vi "green_threshing.vi"(2 "lum":cluster{"Lower value":i32, "Upper value":i32}={"Lower value"=0, "Upper value"=255}, 4 "sat":cluster{"Lower value":i32, "Upper value":i32}={"Lower value"=0, "Upper value"=255}, 5 "hue":cluster{"Lower value":i32, "Upper value":i32}={"Lower value"=50, "Upper value"=102}, 6 "error in (no error)":errorcluster, 9 "Image Src":T1) -> (0 "error out":errorcluster, 1 "circular particles":dbl[][](array[numeric]), 3 "Image Out":T1(plugin-control))   [LabVIEW 2009]
uses:
  <vilib>/vision/Image Controls.llb/IMAQ Image.ctl
  <vilib>/vision/NI_Vision_Development_Module.lvlib
panel:
  in  "max circularity":dbl=1.095
  out "size(s)":i32[](array[numeric])
  out "Particle Measurements (Pixels)":dbl[][](array[numeric]) format="%.2f"
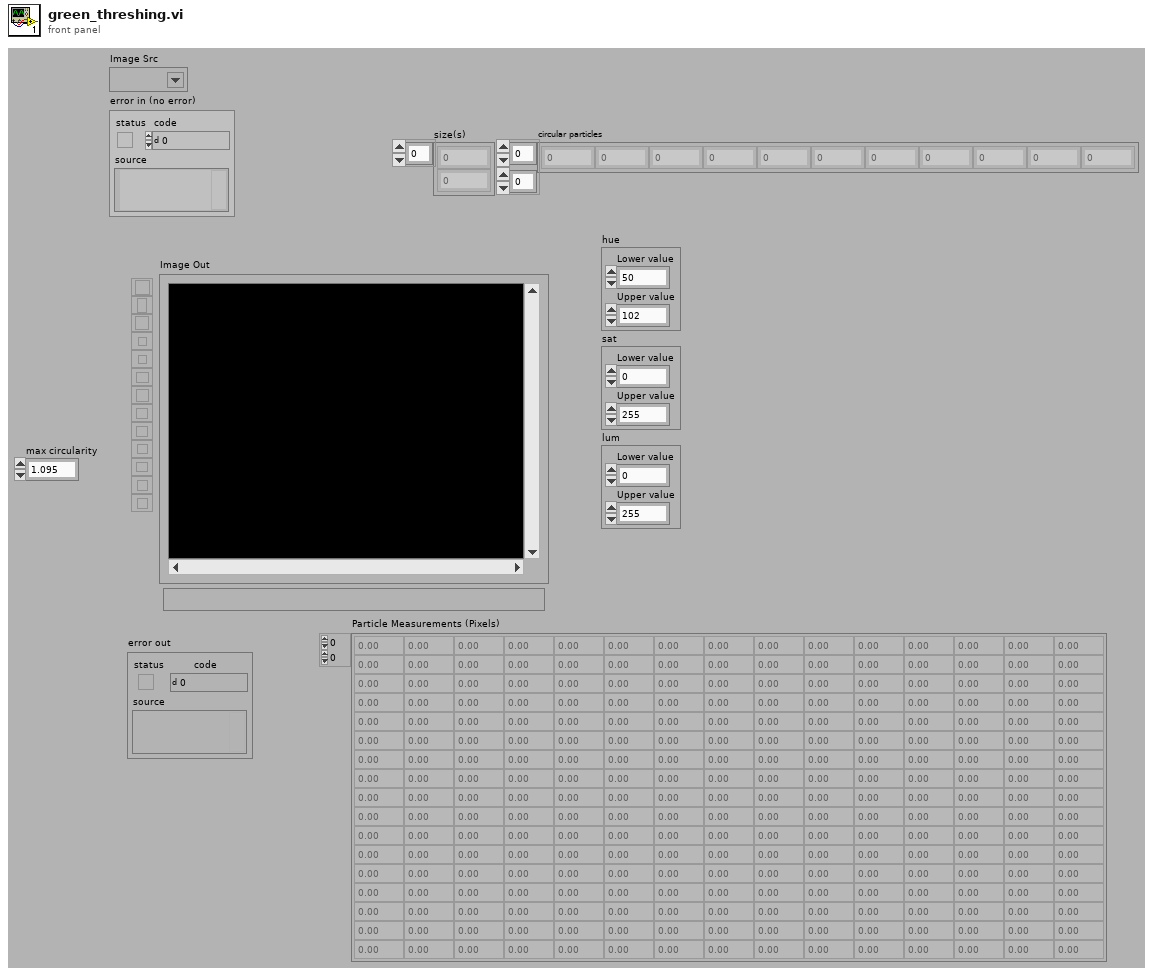
[diagram p1: front panel]
types:
  T1 = typedef "IMAQ Image.ctl" = refnum<image>
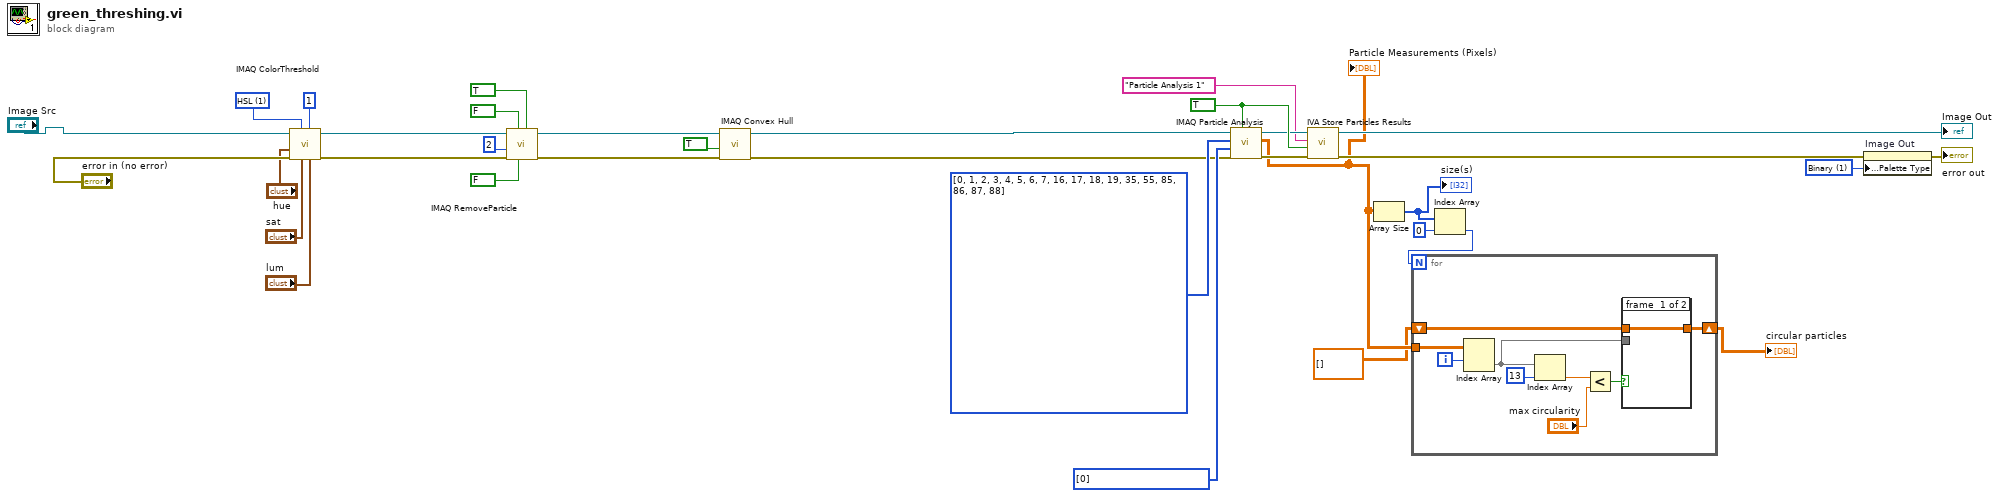
[diagram p0: block diagram]
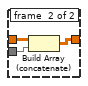
[diagram p2: hidden frame]
diagram:
  w16 = u16 1 items=["RGB", "HSL", "HSV", "HSI"] ("Color Mode")
  w27 = u32 1 items=["Grayscale", "Binary", "Gradient", "Rainbow", "Temperature", "User Defined"] ("Palette")
  w34 = i32[] [0] items=["Center of Mass X", "Center of Mass Y", "First Pixel X", "First Pixel Y", "Bounding Rect Left", "Bounding Rect Top", "Bounding Rect Right", "Bounding Rect Bottom", "Max Feret Diameter Start X", "Max Feret Diameter Start Y", "Max Feret Diameter End X", "Max Feret Diameter End Y", "Max Horiz. Segment Length Left", "Max Horiz. Segment Length Right", "Max Horiz. Segment Length Row", "-", "Bounding Rect Width", "Bounding Rect Height", "Bounding Rect Diagonal", "Perimeter", "Convex Hull Perimeter", "Holes' Perimeter", "Max Feret Diameter", "Equivalent Ellipse Major Axis", "Equivalent Ellipse Minor Axis", "Equivalent Ellipse Minor Axis (Feret)", "Equivalent Rect Long Side", "Equivalent Rect Short Side", "Equivalent Rect Diagonal", "Equivalent Rect Short Side (Feret)", "Average Horiz. Segment Length", "Average Vert. Segment Length", "Hydraulic Radius", "Waddel Disk Diameter", "-", "Area", "Holes' Area", "Particle & Holes' Area", "Convex Hull Area", "Image Area", "-", "Number of Holes", "Number of Horiz. Segments", "Number of Vert. Segments", "-", "Orientation", "Max Feret Diameter Orientation", "-", "% Area/Image Area", "% Area/(Particle & Holes' Area)", "Ratio of Equivalent Ellipse Axes", "Ratio of Equivalent Rect Sides", "-", "Elongation Factor", "Compactness Factor", "Heywood Circularity Factor", "Type Factor", "-", "Sum X", "Sum Y", "Sum XX", "Sum XY", "Sum YY", "Sum XXX", "Sum XXY", "Sum XYY", "Sum YYY", "-", "Moment of Inertia XX", "Moment of Inertia XY", "Moment of Inertia YY", "Moment of Inertia XXX", "Moment of Inertia XXY", "Moment of Inertia XYY", "Moment of Inertia YYY", "Norm. Moment of Inertia XX", "Norm. Moment of Inertia XY", "Norm. Moment of Inertia YY", "Norm. Moment of Inertia XXX", "Norm. Moment of Inertia XXY", "Norm. Moment of Inertia XYY", "Norm. Moment of Inertia YYY", "Hu Moment 1", "Hu Moment 2", "Hu Moment 3", "Hu Moment 4", "Hu Moment 5", "Hu Moment 6", "Hu Moment 7"] ("Real-World Measurements")
  w25 = i32[] [0, 1, 2, 3, 4, 5, 6, 7, 16, 17, 18, 19, 35, 55, 85, 86, 87, 88] items=["Center of Mass X", "Center of Mass Y", "First Pixel X", "First Pixel Y", "Bounding Rect Left", "Bounding Rect Top", "Bounding Rect Right", "Bounding Rect Bottom", "Max Feret Diameter Start X", "Max Feret Diameter Start Y", "Max Feret Diameter End X", "Max Feret Diameter End Y", "Max Horiz. Segment Length Left", "Max Horiz. Segment Length Right", "Max Horiz. Segment Length Row", "-", "Bounding Rect Width", "Bounding Rect Height", "Bounding Rect Diagonal", "Perimeter", "Convex Hull Perimeter", "Holes' Perimeter", "Max Feret Diameter", "Equivalent Ellipse Major Axis", "Equivalent Ellipse Minor Axis", "Equivalent Ellipse Minor Axis (Feret)", "Equivalent Rect Long Side", "Equivalent Rect Short Side", "Equivalent Rect Diagonal", "Equivalent Rect Short Side (Feret)", "Average Horiz. Segment Length", "Average Vert. Segment Length", "Hydraulic Radius", "Waddel Disk Diameter", "-", "Area", "Holes' Area", "Particle & Holes' Area", "Convex Hull Area", "Image Area", "-", "Number of Holes", "Number of Horiz. Segments", "Number of Vert. Segments", "-", "Orientation", "Max Feret Diameter Orientation", "-", "% Area/Image Area", "% Area/(Particle & Holes' Area)", "Ratio of Equivalent Ellipse Axes", "Ratio of Equivalent Rect Sides", "-", "Elongation Factor", "Compactness Factor", "Heywood Circularity Factor", "Type Factor", "-", "Sum X", "Sum Y", "Sum XX", "Sum XY", "Sum YY", "Sum XXX", "Sum XXY", "Sum XYY", "Sum YYY", "-", "Moment of Inertia XX", "Moment of Inertia XY", "Moment of Inertia YY", "Moment of Inertia XXX", "Moment of Inertia XXY", "Moment of Inertia XYY", "Moment of Inertia YYY", "Norm. Moment of Inertia XX", "Norm. Moment of Inertia XY", "Norm. Moment of Inertia YY", "Norm. Moment of Inertia XXX", "Norm. Moment of Inertia XXY", "Norm. Moment of Inertia XYY", "Norm. Moment of Inertia YYY", "Hu Moment 1", "Hu Moment 2", "Hu Moment 3", "Hu Moment 4", "Hu Moment 5", "Hu Moment 6", "Hu Moment 7"] ("Pixel Measurements")
  w33 = TRUE ("Connectivity 4/8 (8)")
  n1 = call "IMAQ ColorThreshold"("Blue or Luma or Val or Inten Range"="lum", "Replace Value"=1, "Green or Sat Range"="sat", "Color Mode"=w16, "error in (no error)"="error in (no error)", "Red or Hue Range"="hue", "Image Src"="Image Src") -> ("error out"=w12:errorcluster, "Image Dst Out"=w7:T1)  [unwired: 1 in, 2 out]
  n2 = call "IMAQ RemoveParticle"("Connectivity 4/8 (8)"=TRUE, "Low Pass/High Pass (Low)"=FALSE, "Square/Hexa (Square)"=FALSE, "error in (no error)"=w12, "Number of Erosion"=2, "Image Src"=w7) -> ("error out"=w6:errorcluster, "Image Dst Out"=w5:T1)  [unwired: 1 in, 3 out]
  n3 = call "IMAQ Convex Hull"("error in (no error)"=w6, "Connectivity 4/8 (8)"=TRUE, "Image Src"=w5) -> ("error out"=w1:errorcluster, "Image Dst Out"=w2:T1)  [unwired: 1 in, 6 out]
  n4 = call "IMAQ Particle Analysis"("Connectivity 4/8 (8)"=w33, "error in (no error)"=w1, "Real-World Measurements"=w34, "Pixel Measurements"=w25, "Image"=w2) -> ("error out"=w30:errorcluster, "Particle Measurements (Pixels)"=w24:dbl[][], "Image Out (duplicate)"=w32:T1)  [unwired: 4 out]
  "Particle Measurements (Pixels)" <- w24
  n5 = call <vilib>:"IVA Store Particles Results.vi"("error in (no error)"=w30, "Connectivity 4/8 (8)"=w33, "Step Name"="Particle Analysis 1", "Image in"=w32) -> ("error out"=w29:errorcluster, "Image dup"=→"Image Out":T1)  [unwired: 6 out]
  n6 = Array Size(array=w24) -> (size(s)=w23:i32[])
  "size(s)" <- w23
  n7 = Index Array(array=w23, index=0) -> (element=w21:i32)
  n8 = for {
    N: w21 -> [_]
    tunnel: w24 -> [w43]
    shift-right: [w35] -> w19
    shift-left: dbl[][] [] ("Particle Measurements (Pixels)") -> [w41]
    i -> [w42]
    n9 = Index Array(array=w43, index (row)=w42) -> (element=w36:dbl[])  [unwired: 1 in]
    n10 = Index Array(array=w36, index=13) -> (element=w39:dbl)
    n11 = Less?(x=w39, y="max circularity") -> (x < y?=w37:bool)
    n12 = case shown="True" w37 {
      tunnel: w41 -> [w44 w47]
      tunnel: w36 -> [_ w46]
      tunnel: [w44 w45] -> w35
      frame #0 {
      }
      frame #1 {
        n13 = Build Array (concatenate)(w47, w46) -> (w45:dbl[][])
      }
    }
  }
  "circular particles" <- w19
  n14 = property on="Image Out" class="ImageControl"(error in=w29, "Palette:Palette Type"=w27) -> (error out=→"error out":errorcluster)  [unwired: 1 in, 1 out]
